vi "SVN Status.vi"(8 "error in (no error)":errorcluster) -> (0 "error out":errorcluster, 1 "Version string":string, 2 "Revision":i32, 3 "standard output":string, 4 "Successful Version Check":bool)   [LabVIEW 2011]
uses:
  SVN.ctl
  Folders.ctl
  Design Server.lvlib
panel:
  out "standard error":string
  in  "SVN":T1
  out "string":string
  out "commandline string":string
  in  "initial string":string="The version number of the MathCAD files used to create this design is"
  in  "Repository URL":string="https://forge.cornell.edu/svn/repos/automated_design/Final Designs/"
  in  "command":string="cmd /c svn info"
  in  "working directory":path=path "C:/Program Files/CollabNet/Subversion Client"
  # "cmd /c svn status  --show-updates wc"
  # "$ svn checkout -r 2 file:///var/svn/repos/test mine"
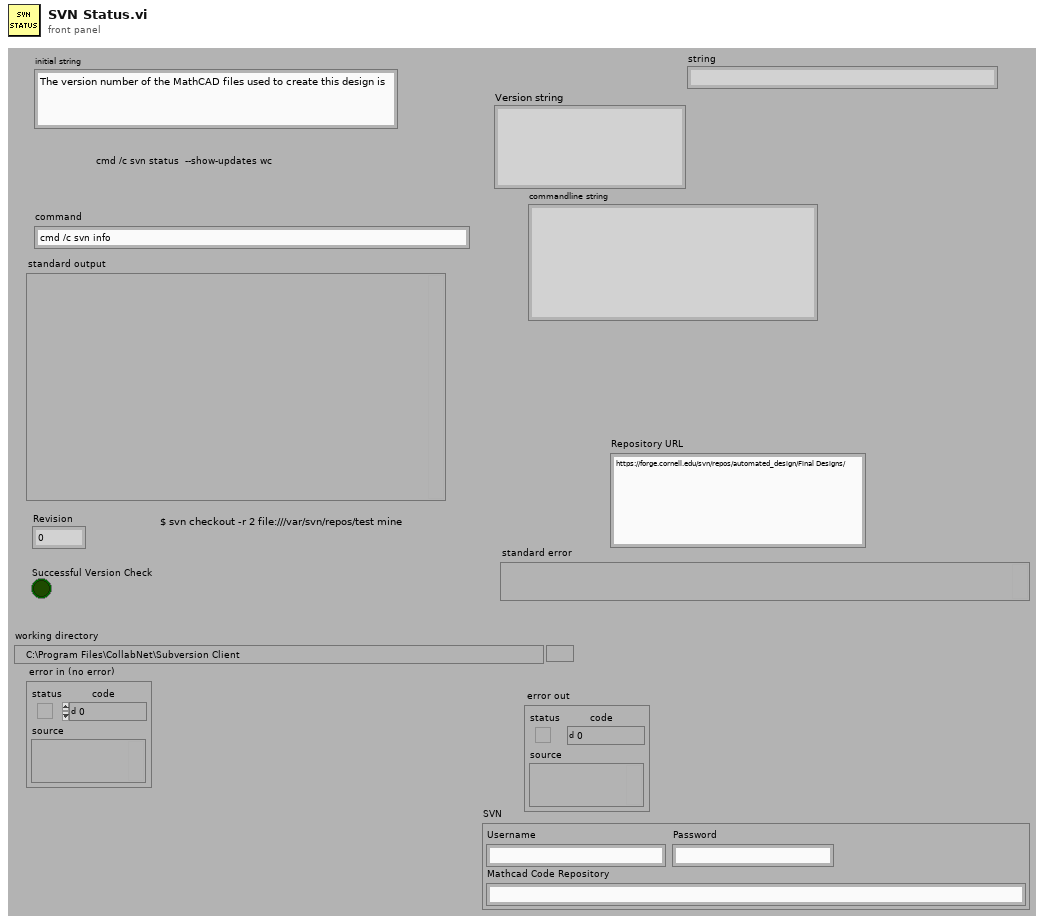
[diagram p1: front panel]
types:
  T1 = typedef "SVN.ctl" = cluster{"Mathcad Code Repository":string, "Username":string, "Password":string}
  T2 = typedef "Design Server.lvlib/Folders.ctl" = enum16{"MathcadMethods", "RequestedDesigns", "CompletedDesigns", "MathcadCode", "CollabnetSVN.exe"}
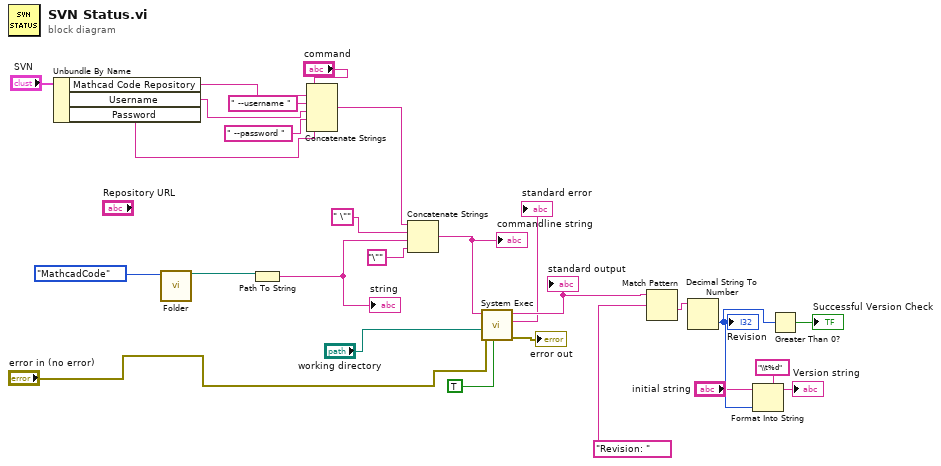
[diagram p0: block diagram]
diagram:
  n1 = Unbundle By Name("SVN") -> ("Mathcad Code Repository"=w7:string, "Username"=w5:string, "Password"=w3:string)
  n2 = call "Folder.vi"("Folders"=Folders."MathcadCode") -> ("FolderPath"=w10:path)  [unwired: 8 in, 2 out]
  n3 = Path To String(path=w10) -> (string=w25:string)
  "string" <- w25
  n4 = Concatenate Strings("command", w7, " --username " ("string"), w5, " --password " ("string"), w3) -> (w1:string)
  n5 = Concatenate Strings(w1, " \"" ("string"), w25, "\"" ("string")) -> (w8:string)
  "commandline string" <- w8
  n6 = call <vilib>:"System Exec.vi"("run minimized? (F)"=TRUE, "error in (no error)"="error in (no error)", "working directory"="working directory", "command line"=w8) -> ("error out"=→"error out":errorcluster, "standard error"=→"standard error":string, "standard output"=w22:string)  [unwired: 4 in, 1 out]
  "standard output" <- w22
  n7 = Match Pattern(string=w22, regular expression="Revision: ") -> (after substring=w20:string)  [unwired: 1 in, 3 out]
  n8 = Decimal String To Number(string=w20) -> (number=w16:i32)  [unwired: 2 in, 1 out]
  "Revision" <- w16
  n9 = Format Into String(format string="\\t%d", initial string="initial string", w16) -> (resulting string=→"Version string":string)  [unwired: 1 in, 1 out]
  n10 = Greater Than 0?(x=w16) -> (x > 0?=→"Successful Version Check":bool)
